vi "Generate Report.vi"() -> ()   [LabVIEW 2020]
uses:
  <vilib>/Utility/sysdir.llb/System Directory Type.ctl
panel:
  in  "Back Square":bool
  in  "Print Report Button":bool
  in  "Paper Size":i32(ring)=2 items=["wdPaper10x14", "wdPaper11x17", "wdPaperLetter", "wdPaperLetterSmall", "wdPaperLegal", "wdPaperExecutive", "wdPaperA3", "wdPaperA4", "wdPaperA4Small", "wdPaperA5", "wdPaperB4", "wdPaperB5", "wdPaperCSheet", "wdPaperDSheet", "wdPaperESheet", "wdPaperFanfoldLegalGerman", "wdPaperFanfoldStdGerman", "wdPaperFanfoldUS", "wdPaperFolio", "wdPaperLedger", "wdPaperNote", "wdPaperQuarto", "wdPaperStatement", "wdPaperTabloid", "wdPaperEnvelope9", "wdPaperEnvelope10", "wdPaperEnvelope11", "wdPaperEnvelope12", "wdPaperEnvelope14", "wdPaperEnvelopeB4", "wdPaperEnvelopeB5", "wdPaperEnvelopeB6", "wdPaperEnvelopeC3", "wdPaperEnvelopeC4", "wdPaperEnvelopeC5", "wdPaperEnvelopeC6", "wdPaperEnvelopeC65", "wdPaperEnvelopeDL", "wdPaperEnvelopeItaly", "wdPaperEnvelopeMonarch", "wdPaperEnvelopePersonal", "wdPaperCustom"]
  out "Status":string
  out "COLHEADERS":string[](array[string])
  out "data":string[][](array[string])
  out "Generate docx and pdf":bool
  in  "DATE COLUMN":string(combo)
  in  "Record count":bool
  in  "Date range":bool
  in  "Record Limit":i32
  in  "END DATE":timestamp format="%<%.0X %x>T"
  in  "START DATE":timestamp format="%<%.0X %x>T"
  in  "Generate Preview":bool
  in  "stop":bool
  in  "Preview":refnum<k7>(container)
  in  "Dataset":string(combo)
  in  "Tempate":string(combo)
  # "GENERATE REPORT"
  # "PREVIEW"
  # "TEMPLATE"
  # "DATASET"
  # "DATE RANGE"
  # "START DATE"
  # "END DATE"
  # "DATE COLUMN"
  # "RECORDS COUNT"
  # "PAPER SIZE"
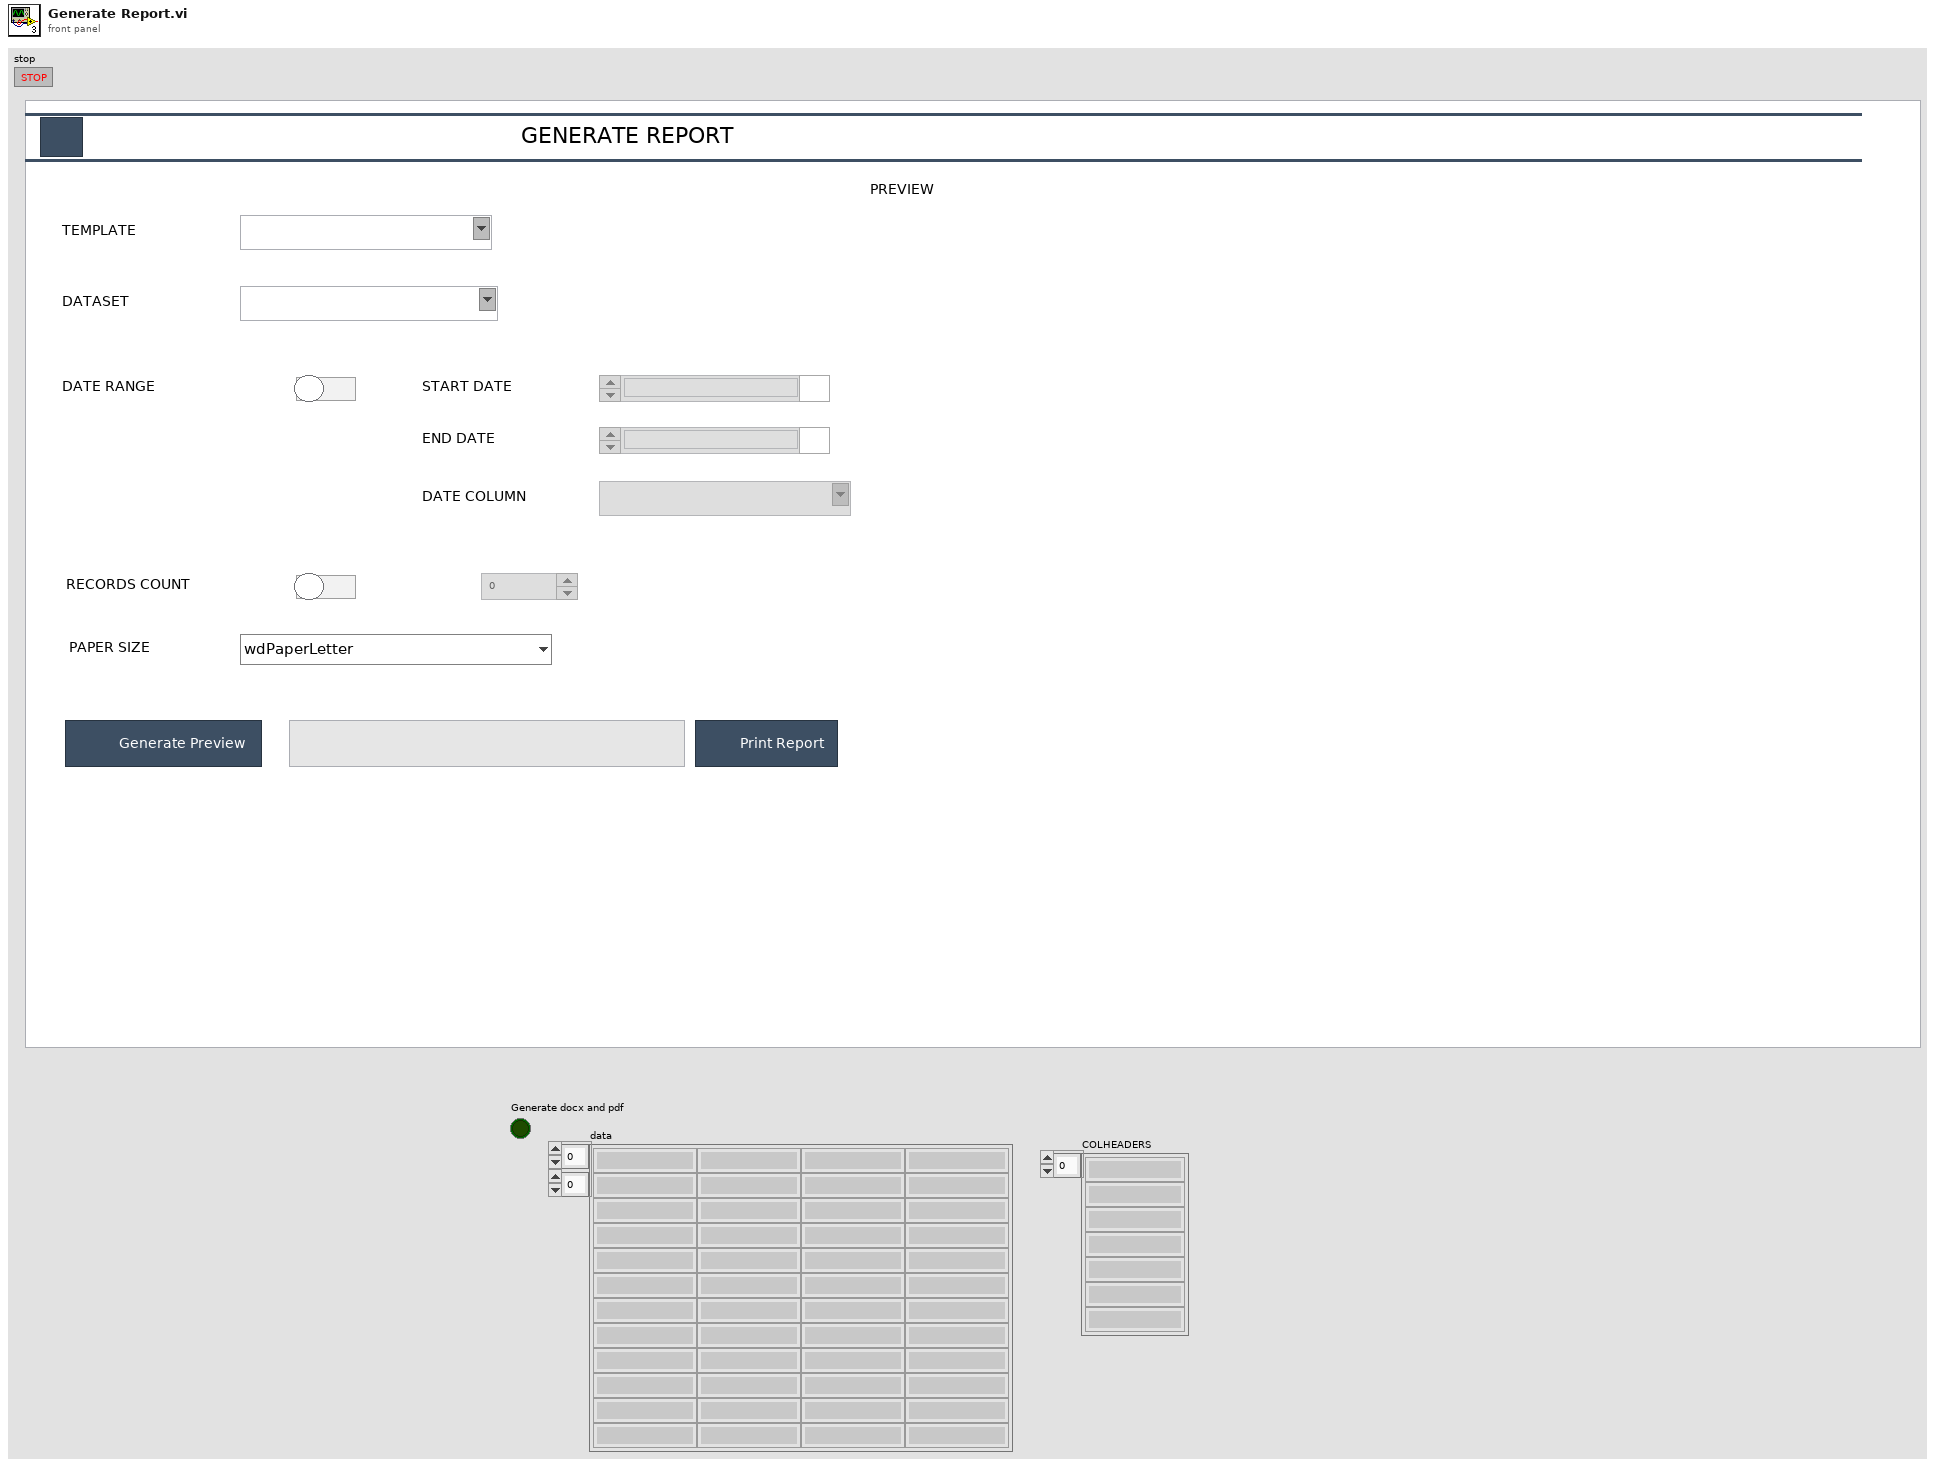
[diagram p1: front panel]
types:
  T1 = typedef "System Directory Type.ctl" = i32
  T2 = enum8{"Enabled", "Disabled", "Disabled and Grayed Out"}
  T3 = cluster{"Query":string, "DB Type":string, "Data Source name":string}
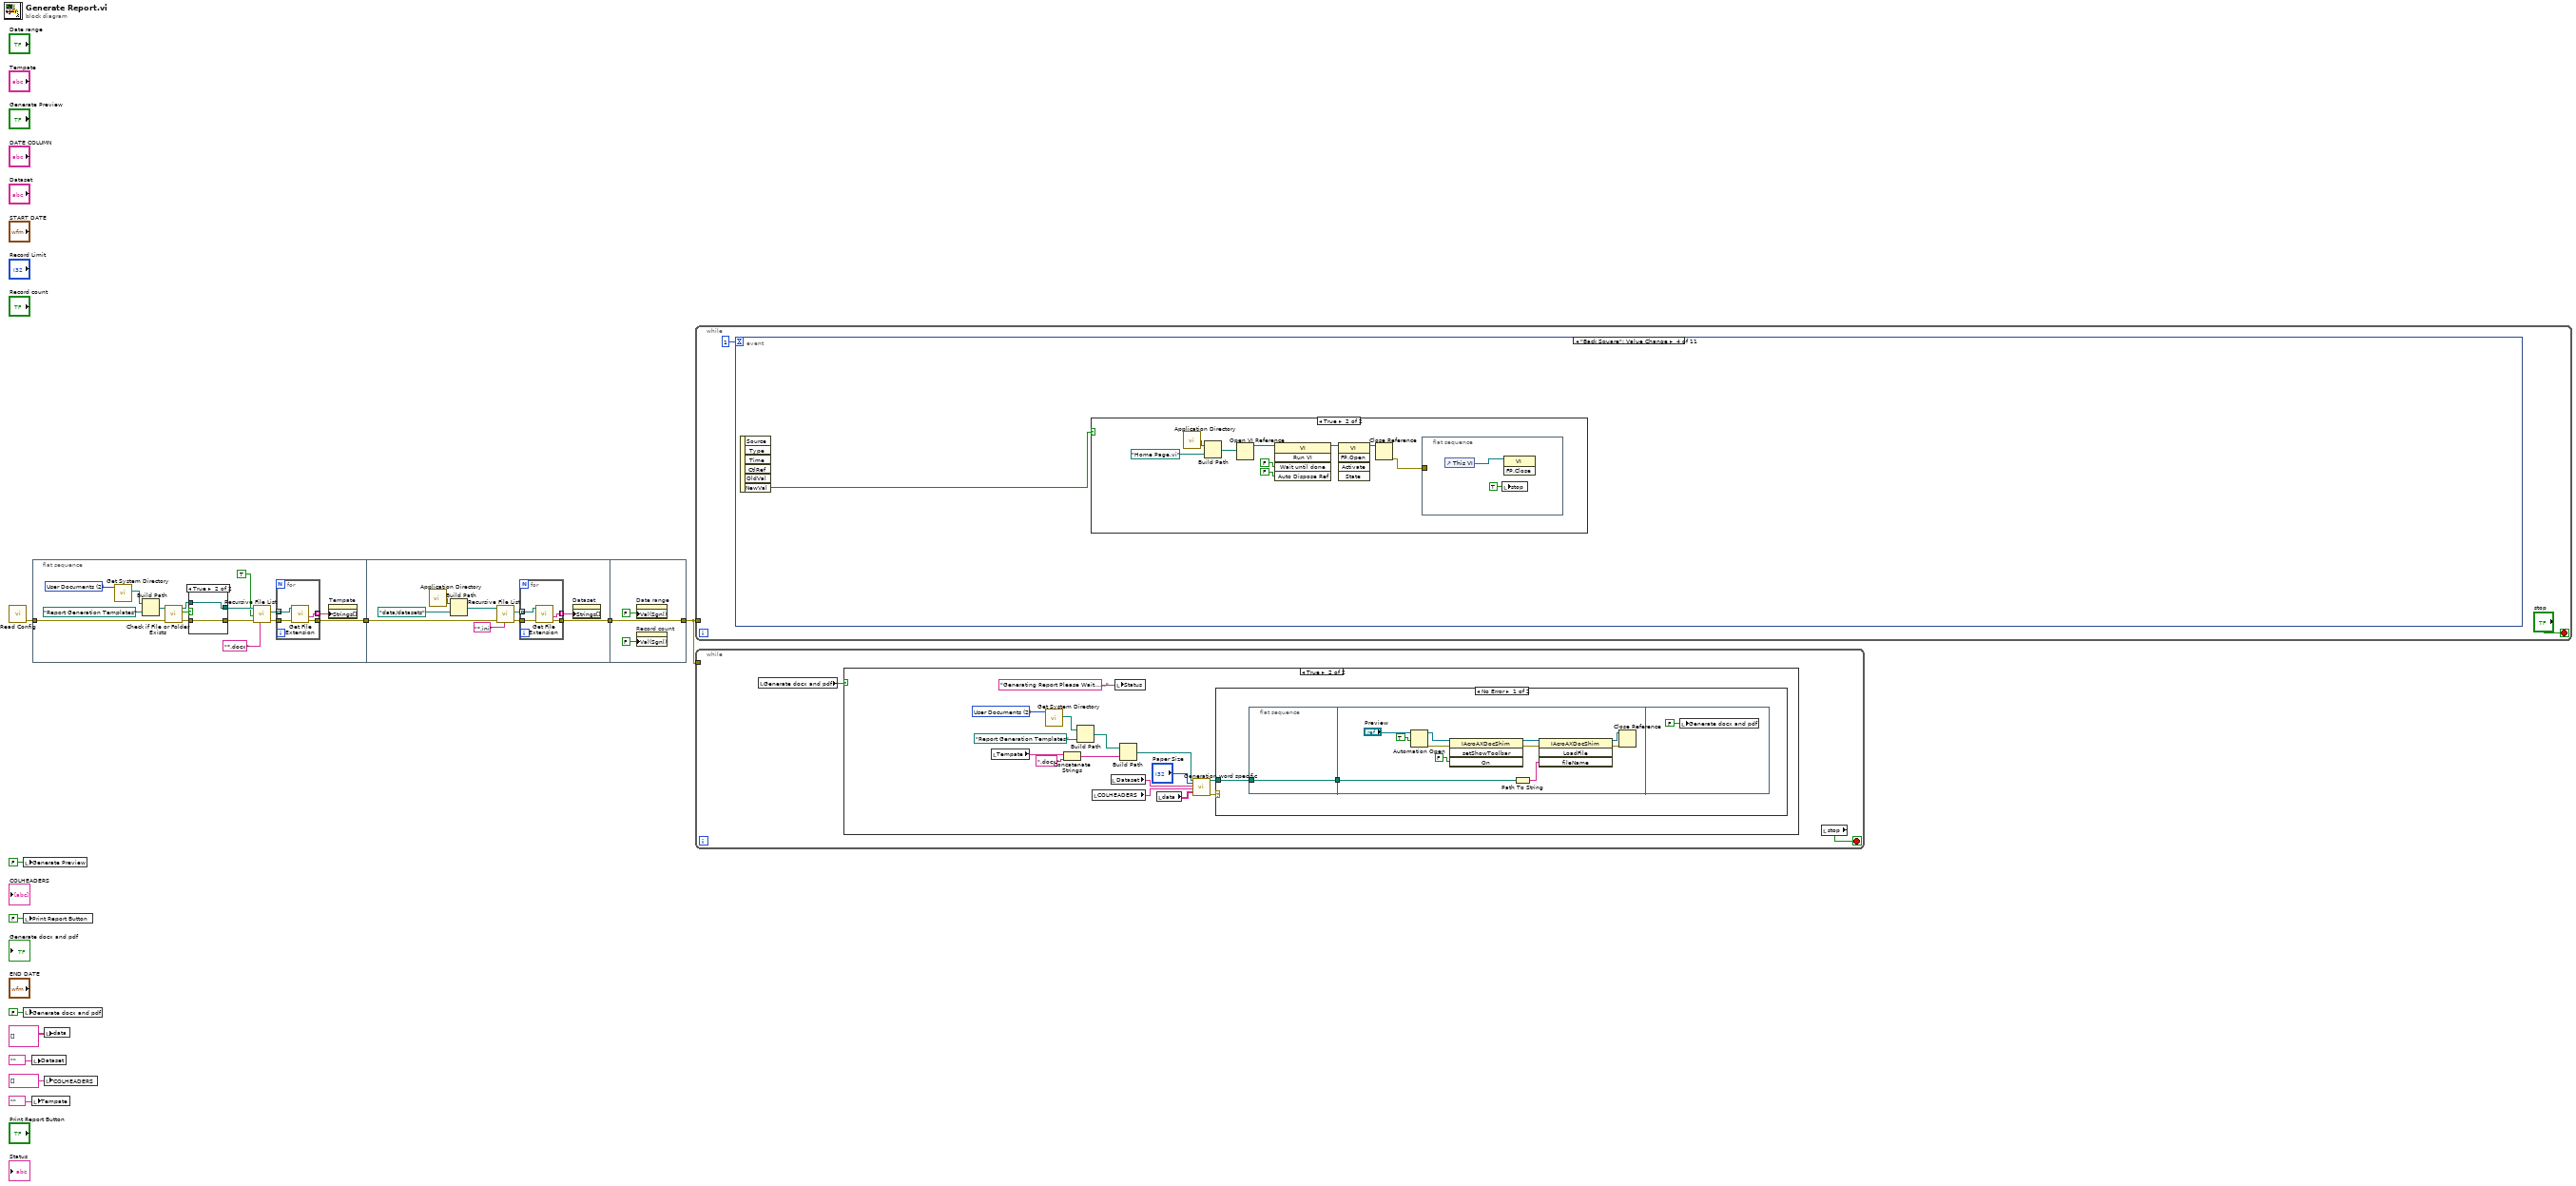
[diagram p0: block diagram]
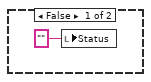
[diagram p2: hidden frame]
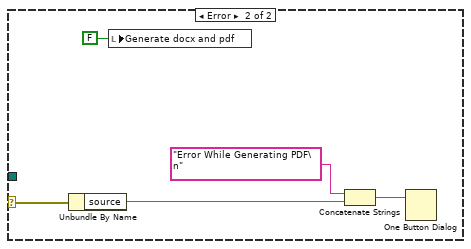
[diagram p3: hidden frame]
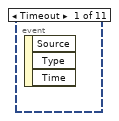
[diagram p4: hidden frame]
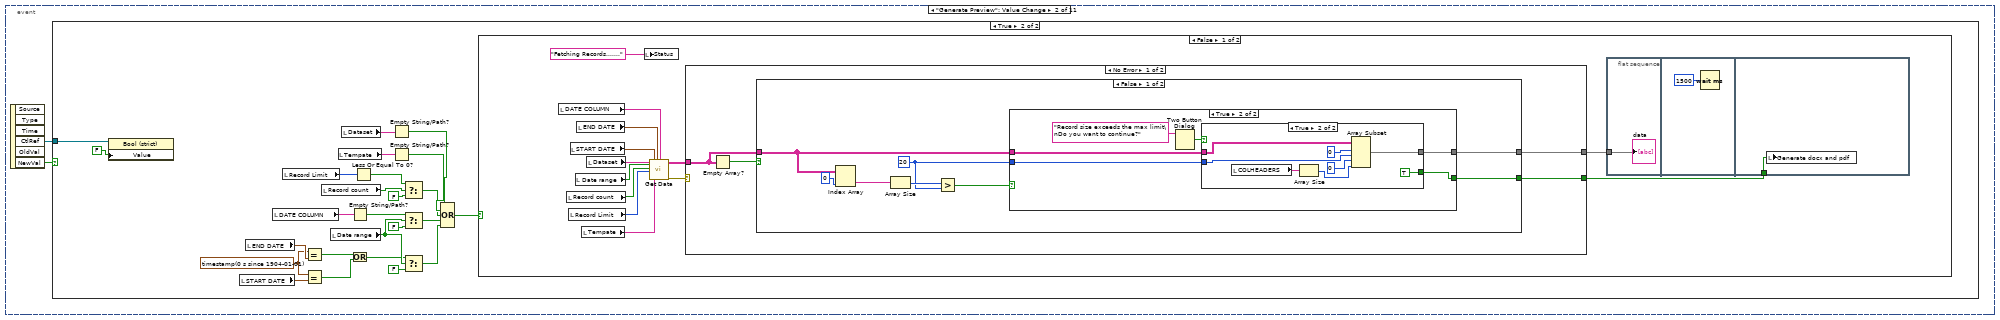
[diagram p5: hidden frame]
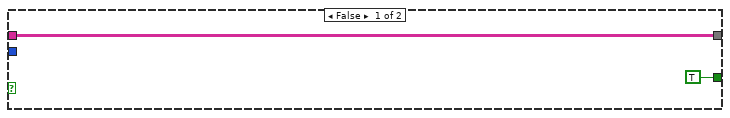
[diagram p7: hidden frame]
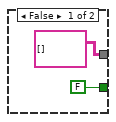
[diagram p8: hidden frame]
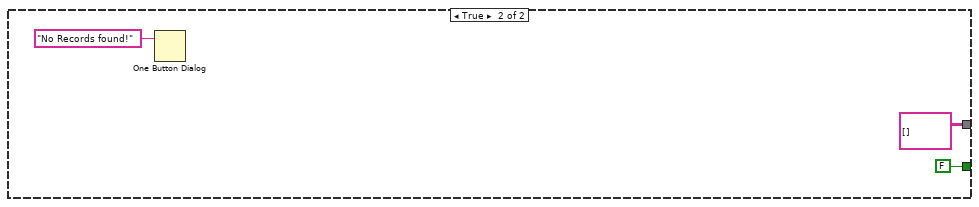
[diagram p9: hidden frame]
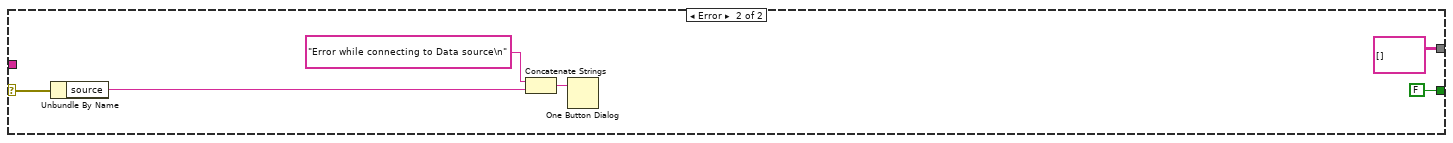
[diagram p10: hidden frame]
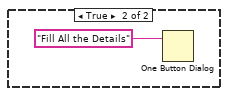
[diagram p11: hidden frame]
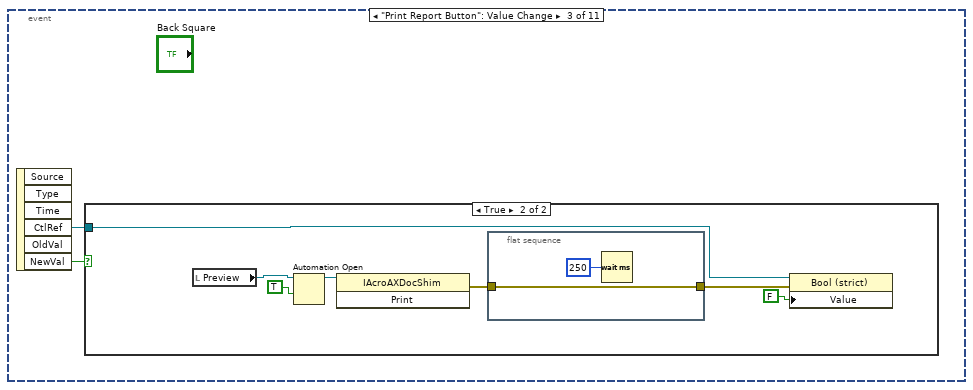
[diagram p12: hidden frame]
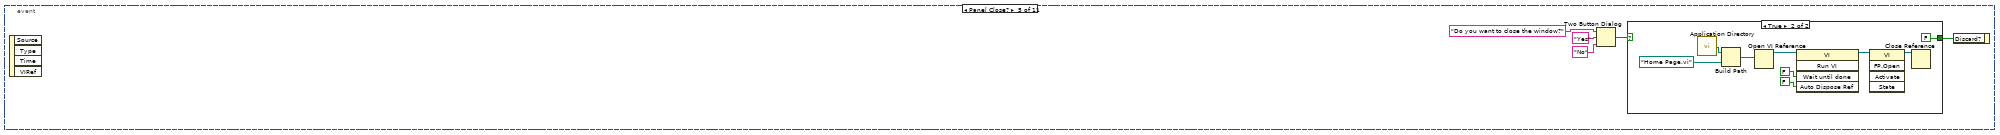
[diagram p15: hidden frame]
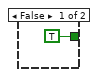
[diagram p16: hidden frame]
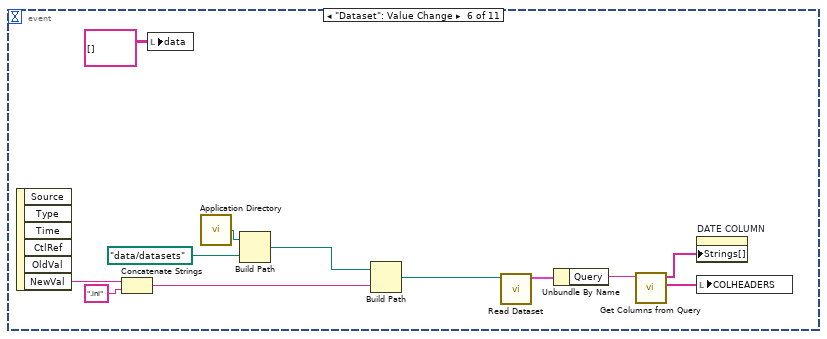
[diagram p17: hidden frame]
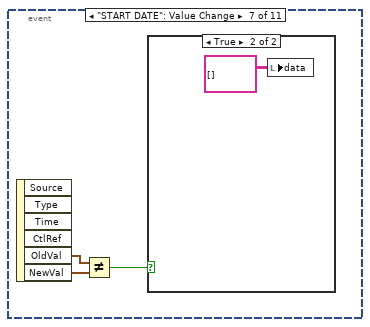
[diagram p18: hidden frame]
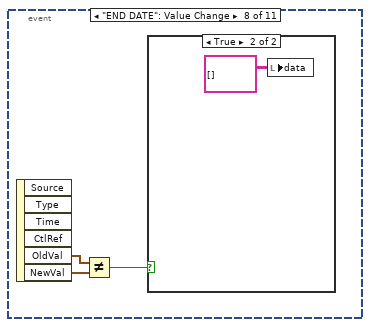
[diagram p20: hidden frame]
diagram:
  n1 = call "Read Config.vi"() -> ("error out"=w11:errorcluster)  [unwired: 10 in, 1 out]
  n2 = local write "Generate Preview"(FALSE ("Generate Preview")) -> ()
  n3 = local write "Print Report Button"(FALSE ("Print Report Button")) -> ()
  n4 = local write "Generate docx and pdf"(FALSE ("Generate docx and pdf")) -> ()
  n5 = local write "Dataset"("" ("Dataset")) -> ()
  n6 = local write "Tempate"("" ("Tempate")) -> ()
  n7 = flat-sequence {
    tunnel: w11 -> [w23]
    tunnel: [w13] -> w10
    tunnel: w10 -> [w42]
    tunnel: [w38] -> w9
    tunnel: [w53] -> w3
    tunnel: w9 -> [w53]
    frame #0 {
      w27 = T1 2 items=["User Home"=0, "User Desktop"=1, "User Documents"=2, "User Application Data"=3, "User Preferences"=4, "User Temporary"=5, "Public Documents"=6, "Public Application Data"=7, "Public Preferences"=8, "Public Cache"=13, "System Core Libraries"=9, "System Installed Libraries"=10, "Application Files"=11, "Boot Volume Root"=12] ("system directory type")
      n8 = call <vilib>:"Get System Directory.vi"("system directory type"=w27) -> ("system directory"=w26:path)  [unwired: 10 in]
      n9 = Build Path(base path=w26, name or relative path=path "Report Generation Templates") -> (appended path=w24:path)
      n10 = call <vilib>:"Check if File or Folder Exists.vi"("error in (no error)"=w23, "path"=w24) -> ("error out"=w20:errorcluster, "file or folder exists?"=w22:bool, "dup path"=w21:path)  [unwired: 7 in]
      n11 = case shown="True" w22 {
        tunnel: w21 -> [w35 w37]
        tunnel: w20 -> [w34 w36]
        tunnel: [w33 w36] -> w18
        tunnel: [w32 w37] -> w19
        frame False {
          n12 = Create Folder(path (use dialog)=w35, error in=w34) -> (created path=w32:path, error out=w33:errorcluster)  [unwired: 1 in, 1 out]
        }
        frame True {
        }
      }
      n13 = call <vilib>:"Recursive File List.vi"("pattern"="*.docx", "error in (no error)"=w18, "Continue Recursing on Error? (F)"=TRUE, "Folder Path"=w19) -> ("error out"=w16:errorcluster, "All Files in Dir"=w14:path[])  [unwired: 3 in, 3 out]
      n14 = for {
        tunnel: w16 -> [w30]
        tunnel: w14 -> [w31] mode=indexing
        tunnel: [w29] -> w15 mode=indexing
        tunnel: [w28] -> w13
        n15 = call <vilib>:"Get File Extension.vi"("error in (no error)"=w30, "file"=w31) -> ("error out"=w28:errorcluster, "filename without extension"=w29:string)  [unwired: 5 in, 3 out]
      }
      n16 = property on="Tempate" class="CmbBox"("Strings[]"=w15) -> ()  [unwired: 2 in, 2 out]
    }
    frame #1 {
      n17 = call <vilib>:"Application Directory.vi"() -> ("Application Directory"=w46:path)
      n18 = Build Path(base path=w46, name or relative path=path "data/datasets") -> (appended path=w44:path)
      n19 = call <vilib>:"Recursive File List.vi"("pattern"="*.ini", "error in (no error)"=w42, "Folder Path"=w44) -> ("error out"=w40:errorcluster, "All Files in Dir"=w41:path[])  [unwired: 4 in, 3 out]
      n20 = for {
        tunnel: w40 -> [w49]
        tunnel: w41 -> [w50] mode=indexing
        tunnel: [w48] -> w39 mode=indexing
        tunnel: [w47] -> w38
        n21 = call <vilib>:"Get File Extension.vi"("error in (no error)"=w49, "file"=w50) -> ("error out"=w47:errorcluster, "filename without extension"=w48:string)  [unwired: 5 in, 3 out]
      }
      n22 = property on="Dataset" class="CmbBox"("Strings[]"=w39) -> ()  [unwired: 2 in, 2 out]
    }
    frame #2 {
      n23 = property on="Date range" class="Bool (strict)"("Val(Sgnl)"=FALSE ("Value (Signaling)")) -> ()  [unwired: 2 in, 2 out]
      n24 = property on="Record count" class="Bool (strict)"("Val(Sgnl)"=FALSE ("Value (Signaling)")) -> ()  [unwired: 2 in, 2 out]
    }
  }
  n25 = local write "data"(string[][] [] ("data")) -> ()
  n26 = local write "COLHEADERS"(string[] [] ("COLHEADERS")) -> ()
  n27 = while {
    tunnel: w3 -> [_]
    stop <- "stop" stop-if-true
    n28 = event shown="[3] \"Back Square\": Value Change" {
      selector: _ -> [_ _ _ _ _ _ _ _ _ _ _]
      dyn-events: _ -> [_ _ _ _ _ _ _ _ _ _ _]
      timeout: 1 -> [_ _ _ _ _ _ _ _ _ _ _]
      event Timeout {
        n29 = event-data() -> ()  [unwired: 1 in, 3 out]
      }
      event "Generate Preview": Value Change {
        n30 = event-data() -> ("CtlRef"=w56:refnum<vi>, "NewVal"=w57:bool)  [unwired: 1 in, 4 out]
        n31 = case shown="True" w57 {
          tunnel: w56 -> [_ w59]
          frame False {
          }
          frame True {
            w67 = timestamp(0 s since 1904-01-01) ("END DATE")
            n32 = property class="Bool (strict)"(reference=w59, "Value"=FALSE) -> ()  [unwired: 1 in, 2 out]
            n33 = local read "START DATE"() -> (w66:timestamp)
            n34 = local read "END DATE"() -> (w68:timestamp)
            n35 = local read "DATE COLUMN"() -> (w72:string)
            n36 = local read "Record Limit"() -> (w74:i32)
            n37 = Equal?(x=w67, y=w68) -> (x = y?=w64:bool)
            n38 = Equal?(x=w67, y=w66) -> (x = y?=w65:bool)
            n39 = local read "Record count"() -> (w77:bool)
            n40 = local read "Date range"() -> (w63:bool)
            n41 = local read "Tempate"() -> (w82:string)
            n42 = local read "Dataset"() -> (w78:string)
            n43 = Empty String/Path?(string/path=w72) -> (empty?=w71:bool)
            n44 = Or(x=w64, y=w65) -> (x .or. y?=w62:bool)
            n45 = Less Or Equal To 0?(x=w74) -> (x <= 0?=w73:bool)
            n46 = Empty String/Path?(string/path=w78) -> (empty?=w81:bool)
            n47 = Empty String/Path?(string/path=w82) -> (empty?=w80:bool)
            n48 = Select(t=w73, s=w77, f=FALSE) -> (s? t:f=w75:bool)
            n49 = Select(t=w71, s=w63, f=FALSE) -> (s? t:f=w69:bool)
            n50 = Select(t=w62, s=w63, f=FALSE) -> (s? t:f=w60:bool)
            n51 = Compound Arithmetic op=OR(w81, w80, w75, w69, w60) -> (w79:bool)
            n52 = case shown="False" w79 {
              frame False {
                n53 = local read "DATE COLUMN"() -> (w92:string)
                n54 = local read "Record count"() -> (w90:bool)
                n55 = local read "Record Limit"() -> (w89:i32)
                n56 = local read "START DATE"() -> (w94:timestamp)
                n57 = local read "Date range"() -> (w91:bool)
                n58 = local read "END DATE"() -> (w93:timestamp)
                n59 = local read "Tempate"() -> (w88:string)
                n60 = local read "Dataset"() -> (w95:string)
                n61 = local write "Status"("Fetching Records......." ("Status")) -> ()
                n62 = call "Get Data.vi"("Dataset name"=w95, "Date range"=w91, "Record count"=w90, "Record Limit"=w89, "START DATE"=w94, "Template"=w88, "END DATE"=w93, "Date Column"=w92) -> ("data"=w85:string[][], "error out"=w87:errorcluster)  [unwired: 10 in]
                n63 = case shown="No Error" w87 {
                  selector: w87 -> [_ w137]
                  tunnel: [w102 string[][] [] ("data")] -> w86
                  tunnel: w85 -> [w100 _]
                  tunnel: [w101 FALSE ("Value (Signaling)")] -> w84
                  frame No Error {
                    n64 = Empty Array?(array=w100) -> (empty?=w99:bool)
                    n65 = case shown="False" w99 {
                      tunnel: [w106 string[][] [] ("data")] -> w102
                      tunnel: [w105 FALSE ("Value (Signaling)")] -> w101
                      tunnel: w100 -> [w103 _]
                      frame False {
                        w104 = 20 ("y")
                        n66 = Index Array(array=w103, index (col)=0 ("disabled index (col)")) -> (element=w109:string[])  [unwired: 1 in]
                        n67 = Array Size(array=w109) -> (size(s)=w108:i32)
                        n68 = Greater?(x=w108, y=w104) -> (0:w107:bool)
                        n69 = case shown="True" w107 {
                          tunnel: w103 -> [w112 w116]
                          tunnel: [w112 w115] -> w106
                          tunnel: [TRUE ("Value (Signaling)") w114] -> w105
                          tunnel: w104 -> [_ w113]
                          frame False {
                          }
                          frame True {
                            n70 = Two Button Dialog(message="Record size exceeds the max limit\nDo you want to continue?") -> (T button?=w117:bool)  [unwired: 2 in]
                            n71 = case shown="True" w117 {
                              tunnel: w116 -> [_ w128]
                              tunnel: [string[][] [] w125] -> w115
                              tunnel: [FALSE ("Value (Signaling)") TRUE ("Value (Signaling)")] -> w114
                              tunnel: w113 -> [_ w121]
                              frame False {
                              }
                              frame True {
                                n72 = local read "COLHEADERS"() -> (w126:string[])
                                n73 = Array Size(array=w126) -> (size(s)=w123:i32)
                                n74 = Array Subset(array=w128, index (row)=0 ("index"), length (row)=w121, index (col)=0 ("index"), length (col)=w123) -> (w125:string[][])
                              }
                            }
                          }
                        }
                      }
                      frame True {
                        n75 = One Button Dialog(message="No Records found!") -> ()  [unwired: 1 in, 1 out]
                      }
                    }
                  }
                  frame Error {
                    n76 = Unbundle By Name(w137) -> ("source"=w135:string)
                    n77 = Concatenate Strings("Error while connecting to Data source\n" ("string"), w135) -> (w134:string)
                    n78 = One Button Dialog(message=w134) -> ()  [unwired: 1 in, 1 out]
                  }
                }
                n79 = flat-sequence {
                  tunnel: w86 -> [w96]
                  tunnel: w84 -> [w98]
                  frame #0 {
                    "data" <- w96
                  }
                  frame #1 {
                    n80 = Wait (ms)(milliseconds to wait=u32 1500) -> ()  [unwired: 1 out]
                  }
                  frame #2 {
                    n81 = local write "Generate docx and pdf"(w98) -> ()
                  }
                }
              }
              frame True {
                n82 = One Button Dialog(message="Fill All the Details") -> ()  [unwired: 1 in, 1 out]
              }
            }
          }
        }
      }
      event "Print Report Button": Value Change {
        n83 = event-data() -> ("CtlRef"=w139:refnum<vi>, "NewVal"=w140:bool)  [unwired: 1 in, 4 out]
        n84 = case shown="True" w140 {
          tunnel: w139 -> [_ w144]
          frame False {
          }
          frame True {
            n85 = local read "Preview"() -> (w146:refnum<k7>)
            n86 = Automation Open(Automation Refnum=w146, 9:TRUE ("open new instance (false)")) -> (Automation Refnum=w145:refnum<k7>)  [unwired: 2 in, 1 out]
            n87 = invoke class="IAcroAXDocShim" method="Print"(reference=w145) -> (error out=w141:errorcluster)  [unwired: 2 in, 2 out]
            n88 = flat-sequence {
              tunnel: [w149] -> w142
              tunnel: w141 -> [w149]
              frame #0 {
                n89 = Wait (ms)(milliseconds to wait=u32 250) -> ()  [unwired: 1 out]
              }
            }
            n90 = property class="Bool (strict)"(reference=w144, error in=w142, "Value"=FALSE) -> ()  [unwired: 2 out]
          }
        }
      }
      event "Back Square": Value Change {
        n91 = event-data() -> ("NewVal"=w150:bool)  [unwired: 1 in, 5 out]
        n92 = case shown="True" w150 {
          frame False {
          }
          frame True {
            n93 = call <vilib>:"Application Directory.vi"() -> ("Application Directory"=w159:path)
            n94 = Build Path(base path=w159, name or relative path=path "Home Page.vi") -> (appended path=w157:path)
            n95 = Open VI Reference(vi path=w157) -> (vi reference=w156:refnum<vi>)  [unwired: 5 in, 1 out]
            n96 = invoke class="VI" method="Run VI"(reference=w156, "Wait until done"=FALSE ("Wait Until Done"), "Auto Dispose Ref"=FALSE ("Auto Dispose Reference")) -> (reference out=w155:refnum<vi>)  [unwired: 2 in, 4 out]
            n97 = invoke class="VI" method="FP.Open"(reference=w155) -> (reference out=w152:refnum<vi>)  [unwired: 4 in, 4 out]
            n98 = Close Reference(reference=w152) -> (error out=w151:errorcluster)  [unwired: 1 in]
            n99 = flat-sequence {
              tunnel: w151 -> [_]
              frame #0 {
                n100 = control-ref of="This VI"() -> (w161:refnum<vi>)
                n101 = local write "stop"(TRUE ("stop")) -> ()
                n102 = invoke class="VI" method="FP.Close"(reference=w161) -> ()  [unwired: 2 in, 3 out]
              }
            }
          }
        }
      }
      event Panel Close? {
        n103 = event-data() -> ()  [unwired: 1 in, 4 out]
        n104 = Two Button Dialog(message="Do you want to close the window?", 1:"No" ("F button name (\"Cancel\")"), 2:"Yes" ("T button name (\"OK\")")) -> (T button?=w163:bool)
        n105 = case shown="True" w163 {
          tunnel: [TRUE ("Discard?") FALSE ("Discard?")] -> w162
          frame False {
          }
          frame True {
            n106 = call <vilib>:"Application Directory.vi"() -> ("Application Directory"=w175:path)
            n107 = Build Path(base path=w175, name or relative path=path "Home Page.vi") -> (appended path=w173:path)
            n108 = Open VI Reference(vi path=w173) -> (vi reference=w172:refnum<vi>)  [unwired: 5 in, 1 out]
            n109 = invoke class="VI" method="Run VI"(reference=w172, "Wait until done"=FALSE ("Wait Until Done"), "Auto Dispose Ref"=FALSE ("Auto Dispose Reference")) -> (reference out=w171:refnum<vi>)  [unwired: 2 in, 4 out]
            n110 = invoke class="VI" method="FP.Open"(reference=w171) -> (reference out=w168:refnum<vi>)  [unwired: 4 in, 4 out]
            n111 = Close Reference(reference=w168) -> ()  [unwired: 1 in, 1 out]
          }
        }
        n112 = event-data("Discard?"=w162) -> ()  [unwired: 1 in, 1 out]
      }
      event "Dataset": Value Change {
        n113 = event-data() -> ("NewVal"=w188:string)  [unwired: 1 in, 5 out]
        n114 = Concatenate Strings(w188, ".ini" ("string")) -> (w182:string)
        n115 = local write "data"(string[][] [] ("data")) -> ()
        n116 = call <vilib>:"Application Directory.vi"() -> ("Application Directory"=w186:path)
        n117 = Build Path(base path=w186, name or relative path=path "data/datasets") -> (appended path=w184:path)
        n118 = Build Path(base path=w184, name or relative path=w182) -> (appended path=w181:path)
        n119 = call "Read Dataset.vi"("Saving Path"=w181) -> ("Information"=w180:T3)  [unwired: 9 in, 1 out]
        n120 = Unbundle By Name(w180) -> ("Query"=w179:string)
        n121 = call "Get Columns from Query.vi"("Query"=w179) -> ("COLHEADERS"=w177:string[], "Array"=w187:string[])  [unwired: 8 in, 1 out]
        n122 = property on="DATE COLUMN" class="CmbBox"("Strings[]"=w187) -> ()  [unwired: 2 in, 2 out]
        n123 = local write "COLHEADERS"(w177) -> ()
      }
      event "START DATE": Value Change {
        n124 = event-data() -> ("OldVal"=w191:timestamp, "NewVal"=w190:timestamp)  [unwired: 1 in, 4 out]
        n125 = Not Equal?(x=w191, y=w190) -> (x != y?=w189:bool)
        n126 = case shown="True" w189 {
          frame False {
          }
          frame True {
            n127 = local write "data"(string[][] [] ("data")) -> ()
          }
        }
      }
      event "END DATE": Value Change {
        n128 = event-data() -> ("OldVal"=w195:timestamp, "NewVal"=w194:timestamp)  [unwired: 1 in, 4 out]
        n129 = Not Equal?(x=w195, y=w194) -> (x != y?=w193:bool)
        n130 = case shown="True" w193 {
          frame False {
          }
          frame True {
            n131 = local write "data"(string[][] [] ("data")) -> ()
          }
        }
      }
      event "Record Limit": Value Change {
        n132 = event-data() -> ("OldVal"=w199:i32, "NewVal"=w198:i32)  [unwired: 1 in, 4 out]
        n133 = Not Equal?(x=w199, y=w198) -> (x != y?=w197:bool)
        n134 = case shown="True" w197 {
          frame False {
          }
          frame True {
            n135 = local write "data"(string[][] [] ("data")) -> ()
          }
        }
      }
      event "Date range": Value Change {
        n136 = event-data() -> ("NewVal"=w202:bool)  [unwired: 1 in, 5 out]
        n137 = Select(t=T2."Enabled" ("Disabled"), s=w202, f=T2."Disabled and Grayed Out" ("Disabled")) -> (s? t:f=w201:T2)
        n138 = property on="END DATE" class="AbsTime (strict)"("DisabledEnum"=w201) -> ()  [unwired: 2 in, 2 out]
        n139 = property on="START DATE" class="AbsTime (strict)"("DisabledEnum"=w201) -> ()  [unwired: 2 in, 2 out]
        n140 = property on="DATE COLUMN" class="CmbBox"("DisabledEnum"=w201) -> ()  [unwired: 2 in, 2 out]
      }
      event "Record count": Value Change {
        n141 = event-data() -> ("NewVal"=w206:bool)  [unwired: 1 in, 5 out]
        n142 = Select(t=T2."Enabled" ("Disabled"), s=w206, f=T2."Disabled and Grayed Out" ("Disabled")) -> (s? t:f=w205:T2)
        n143 = property on="Record Limit" class="DigNum (strict)"("DisabledEnum"=w205) -> ()  [unwired: 2 in, 2 out]
      }
    }
  }
  n144 = while {
    tunnel: w3 -> [_]
    stop <- w210 stop-if-true
    n145 = local read "Generate docx and pdf"() -> (w209:bool)
    n146 = case shown="True" w209 {
      frame False {
        n147 = local write "Status"("" ("Status")) -> ()
      }
      frame True {
        w219 = T1 2 items=["User Home"=0, "User Desktop"=1, "User Documents"=2, "User Application Data"=3, "User Preferences"=4, "User Temporary"=5, "Public Documents"=6, "Public Application Data"=7, "Public Preferences"=8, "Public Cache"=13, "System Core Libraries"=9, "System Installed Libraries"=10, "Application Files"=11, "Boot Volume Root"=12] ("system directory type")
        n148 = local read "Tempate"() -> (w223:string)
        n149 = call <vilib>:"Get System Directory.vi"("system directory type"=w219) -> ("system directory"=w220:path)  [unwired: 10 in]
        n150 = Concatenate Strings(w223, ".docx" ("string")) -> (w217:string)
        n151 = Build Path(base path=w220, name or relative path=path "Report Generation Templates") -> (appended path=w218:path)
        n152 = local read "COLHEADERS"() -> (w225:string[])
        n153 = local read "Dataset"() -> (w226:string)
        n154 = local write "Status"("Generating Report Please Wait......" ("Status")) -> ()
        n155 = Build Path(base path=w218, name or relative path=w217) -> (appended path=w216:path)
        n156 = local read "data"() -> (w224:string[][])
        n157 = call "Generation word specific.vi"("Template Path"=w216, "paper size (letter)"="Paper Size", "Data Set Name"=w226, "column headers"=w225, "Table Data"=w224) -> ("Report Saved Path"=w214:path, "error out"=w215:errorcluster)  [unwired: 13 in]
        n158 = case shown="No Error" w215 {
          selector: w215 -> [_ w244]
          tunnel: w214 -> [w228 _]
          frame No Error {
            n159 = flat-sequence {
              tunnel: w228 -> [w229]
              tunnel: [w229] -> w227
              tunnel: w227 -> [w233]
              frame #0 {
              }
              frame #1 {
                n160 = Automation Open(Automation Refnum="Preview", 9:TRUE ("open new instance (false)")) -> (Automation Refnum=w239:refnum<k7>, error out=w240:errorcluster)  [unwired: 2 in]
                n161 = invoke class="IAcroAXDocShim" method="setShowToolbar"(reference=w239, error in=w240, "On"=FALSE) -> (reference out=w237:refnum<k7>, error out=w238:errorcluster)  [unwired: 1 in, 2 out]
                n162 = Path To String(path=w233) -> (string=w232:string)
                n163 = invoke class="IAcroAXDocShim" method="LoadFile"(reference=w237, error in=w238, "fileName"=w232) -> (reference out=w235:refnum<k7>, error out=w236:errorcluster)  [unwired: 1 in, 2 out]
                n164 = Close Reference(reference=w235, error in (no error)=w236) -> ()  [unwired: 1 out]
              }
              frame #2 {
                n165 = local write "Generate docx and pdf"(FALSE ("Generate docx and pdf")) -> ()
              }
            }
          }
          frame Error {
            n166 = Unbundle By Name(w244) -> ("source"=w245:string)
            n167 = local write "Generate docx and pdf"(FALSE ("Generate docx and pdf")) -> ()
            n168 = Concatenate Strings("Error While Generating PDF\n" ("string"), w245) -> (w243:string)
            n169 = One Button Dialog(message=w243) -> ()  [unwired: 1 in, 1 out]
          }
        }
      }
    }
    n170 = local read "stop"() -> (w210:bool)
  }
